vi "set_experiment_state.vi"(8 "error in (no error)":errorcluster, 10 "GLOBAL SETTINGS IN":refnum<notifier>, 11 "EXPERIMENT SETTINGS IN":refnum<notifier>) -> (0 "error out":errorcluster, 2 "GLOBAL SETTINGS OUT":refnum<notifier>, 3 "EXPERIMENT SETTINGS OUT":refnum<notifier>)   [LabVIEW 2013]
uses:
  type_defs/global_settings.ctl
  type_defs/experiment_settings.ctl
  type_defs/experiment_states.ctl
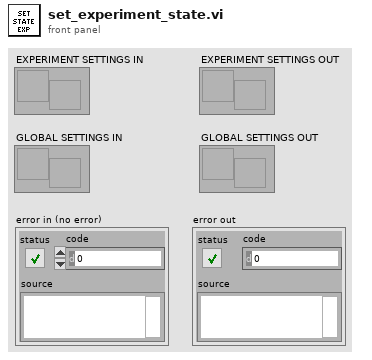
[diagram p1: front panel]
types:
  T1 = typedef "experiment_settings.ctl" = cluster{"fcs file byte offset":i64, "LED Device Handle Out":u32, "START TIME":timestamp, "CURRENT VALVE":u32, "SAMPLE #":i32, "FCS FILE PATH":path, "TIME POINT":i32, "STATE":T2, "TIME TILL SAMPLE":dbl, "DILUTION  TABLE":dbl[][]}
  T2 = typedef "experiment_states.ctl" = enum16{"OUTGROWTH", "INDUCTION", "EXPERIMENT"}
  T3 = typedef "global_settings.ctl" = cluster{"# REACTORS":u32, "17X PORT":i32, "WASTE POSITION ":i32, "SECONDS BETWEEN SAMPLING":dbl, "FACS DIVA DIRECTORY":path, "DATA FILE":path, "REACTORS TO USE":u32[], "PULSE PERIOD":i32, "USE LIGHTS?":bool, "LED FILE":path, "LED CHANNELS":u32[], "PULSE LENGTH":i32, "SUMMARY FILE":path, "OUTGROWTH TIME POINTS":dbl, "SELECTION VALVE PORT":refnum<visa-resource-name>, "HTS PORT":refnum<visa-resource-name>, "DILUTION VOLUME (uL)":i32, "DILUTION FILE":path, "1X PORT":i32}
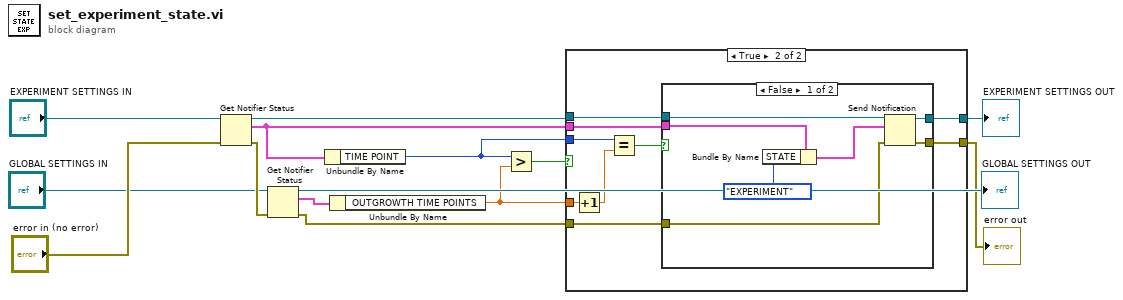
[diagram p0: block diagram]
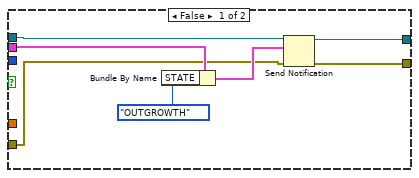
[diagram p2: hidden frame]
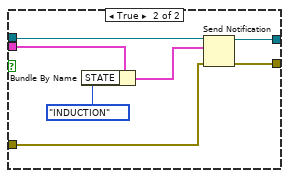
[diagram p3: hidden frame]
diagram:
  n1 = Get Notifier Status(notifier="EXPERIMENT SETTINGS IN", error in (no error)="error in (no error)") -> (notifier out=w12:refnum<notifier>, current notification=w10:T1, error out=w3:errorcluster)  [unwired: 2 out]
  n2 = Get Notifier Status(notifier="GLOBAL SETTINGS IN", error in (no error)=w3) -> (notifier out=→"GLOBAL SETTINGS OUT":refnum<notifier>, current notification=w8:T3, error out=w11:errorcluster)  [unwired: 2 out]
  n3 = Unbundle By Name(w10) -> ("TIME POINT"=w7:i32)
  n4 = Unbundle By Name(w8) -> ("OUTGROWTH TIME POINTS"=w9:dbl)
  n5 = Greater?(x=w7, y=w9) -> (0:w6:bool)
  n6 = case shown="True" w6 {
    tunnel: w7 -> [_ w29]
    tunnel: w9 -> [_ w30]
    tunnel: w10 -> [w18 w26]
    tunnel: w11 -> [w15 w25]
    tunnel: w12 -> [w19 w24]
    tunnel: [w16 w23] -> w1
    tunnel: [w17 w22] -> w13
    frame False {
      n7 = Bundle By Name(cluster=w18, "STATE"=experiment_states."OUTGROWTH") -> (w20:T1)
      n8 = Send Notification(notification=w20, notifier=w19, error in (no error)=w15) -> (notifier out=w17:refnum<notifier>, error out=w16:errorcluster)
    }
    frame True {
      n9 = Increment(x=w30) -> (x+1=w27:dbl)
      n10 = Equal?(x=w29, y=w27) -> (x = y?=w28:bool)
      n11 = case shown="False" w28 {
        tunnel: w26 -> [w34 w44]
        tunnel: w25 -> [w33 w41]
        tunnel: w24 -> [w35 w40]
        tunnel: [w32 w39] -> w23
        tunnel: [w31 w38] -> w22
        frame False {
          n12 = Bundle By Name(cluster=w34, "STATE"=experiment_states."EXPERIMENT") -> (w36:T1)
          n13 = Send Notification(notification=w36, notifier=w35, error in (no error)=w33) -> (notifier out=w31:refnum<notifier>, error out=w32:errorcluster)
        }
        frame True {
          n14 = Bundle By Name(cluster=w44, "STATE"=experiment_states."INDUCTION") -> (w42:T1)
          n15 = Send Notification(notification=w42, notifier=w40, error in (no error)=w41) -> (notifier out=w38:refnum<notifier>, error out=w39:errorcluster)
        }
      }
    }
  }
  "EXPERIMENT SETTINGS OUT" <- w13
  "error out" <- w1
